vi "SW_Combinations.vi"() -> ()   [LabVIEW 2016]
panel:
  in  "SW_Comb":i32[][](array[numeric])
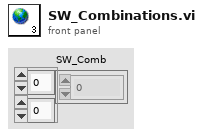
[diagram p1: front panel]
diagram:
